vi "故障码字段定义.vi"(7 "id":u16, 11 "故障代码":u16(ring)) -> (3 "告警信息":T1)   [LabVIEW 2016, in "斯坦道氨氮.lvlib"]
uses:
  Alarm interface/Alarm interface.lvlib
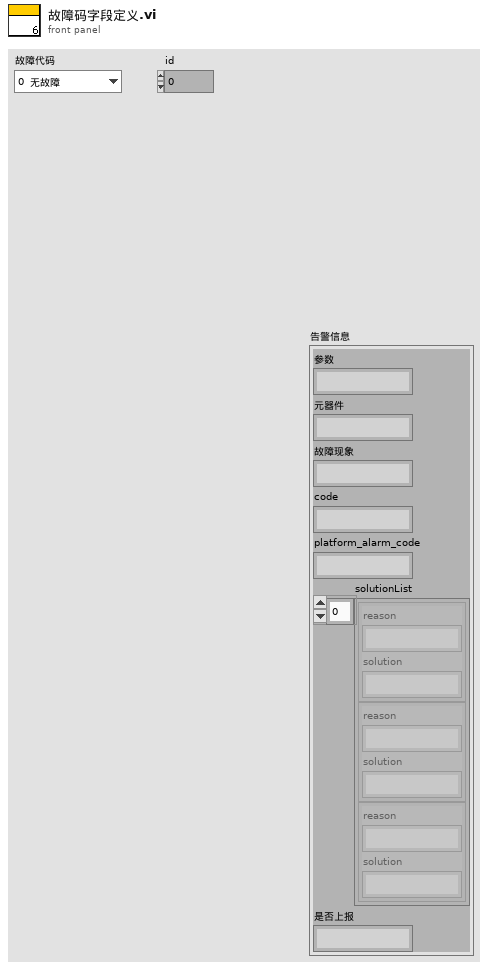
[diagram p1: front panel]
types:
  T1 = typedef "Alarm interface.lvlib/报警短信语音交互.ctl" = cluster{"参数":string, "元器件":string, "故障现象":string, "code":string, "platform_alarm_code":string, "solutionList":cluster{"reason":string, "solution":string}[], "是否上报":string}
  T2 = typedef "Alarm interface.lvlib/map in.ctl" = cluster{"name":string, "CN":string, "FirmwareVersion":string, "code":string}
  T3 = typedef "SingleStepTestV3.lvlib/SingleStepTestV3.lvclass/仪器版本.ctl" = enum16{"V3.1版", "V4版", "V3版", "V4.2版"}
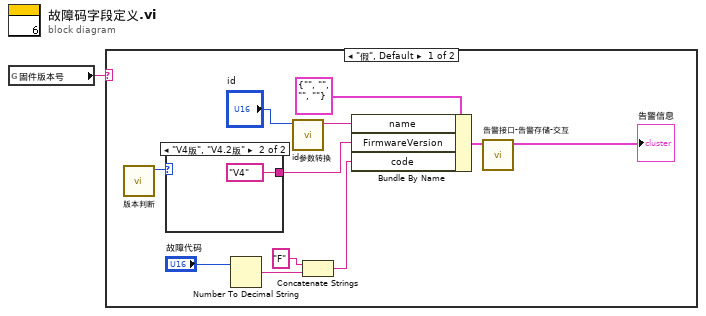
[diagram p0: block diagram]
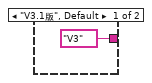
[diagram p2: hidden frame]
diagram:
  n1 = global read "VAR总磷总氮全局变量.vi" "固件版本号"() -> (w1:string)
  n2 = case shown="\"假\", Default" w1 {
    frame "假", Default {
      n3 = call "版本判断.vi"() -> ("仪器版本"=w9:T3)  [unwired: 11 in]
      n4 = case shown="\"V4版\", \"V4.2版\"" w9 {
        tunnel: ["V3" ("equipVersion") "V4" ("equipVersion")] -> w8
        frame "V3.1版", Default {
        }
        frame "V4版", "V4.2版" {
        }
      }
      n5 = Number To Decimal String(number="故障代码") -> (decimal integer string=w6:string)  [unwired: 1 in]
      n6 = call "id参数转换.vi"("id"="id") -> ("table输出"=w10:string)  [unwired: 9 in, 1 out]
      n7 = Concatenate Strings("F" ("字符串"), w6) -> (w4:string)
      n8 = Bundle By Name(cluster=T2 {"name"="", "CN"="", "FirmwareVersion"="", "code"=""} ("map in"), "name"=w10, "FirmwareVersion"=w8, "code"=w4) -> (w2:T2)
      n9 = call "告警接口-告警存储-交互.vi"("map in"=w2) -> ("data"=→"告警信息":T1)  [unwired: 10 in]
    }
    frame "" {
    }
  }
